vi "2.1 Interpret NMEA Sentence.vi"(11 "NMEA Sentence":string) -> ()   [LabVIEW 2011]
doc: "Interprets the NMEA 0813 sentences that we are using from our Airmar PB200 WeatherStation sensor.\nBy Jaime McCandless\nTODO: finish implementing NMEA sentences"
uses:
  <vilib>/regexp/Match Regular Expression.xnode
panel:
  out "Tab Control":enum32{"GPRMC", "GPGGA", "GPGLL"}(tab)
  out "UTC Time":timestamp
  out "Local Time":timestamp
  out "Lattitude (ddmm.mmmm)":dbl format="%_8g"
  out "Lattitude North/South":string
  out "Longitude (ddmm.mmmm)":dbl format="%_8g"
  out "Longitude East/West":string
  out "Speed over ground (knots)":dbl format="%_3g"
  out "Course over ground (degrees)":dbl format="%_4g"
  out "Magnetic Variation (degrees)":dbl format="%_4g"
  out "Variation East/West":string
  out "GPS (RMC) Data":T1 {"Course over ground (degrees)" format="%#.6g"; "Speed over ground (knots)" format="%#.6g"; "Magnetic Variation (degrees)" format="%#.6g"; "Longitude (ddmm.mmmm)" format="%#.6g"; "Lattitude (ddmm.mmmm)" format="%#.6g"}
  in  "UTC Time Zone":i32=-5
  out "GPS Data Valid?":bool
  out "UTC Time":timestamp
  out "Local Time":timestamp
  out "Lattitude (ddmm.mmmm)":dbl format="%_8g"
  out "Longitude (ddmm.mmmm)":dbl format="%_8g"
  out "Latitude North/South":string
  out "Longitude East/West":string
  in  "UTC Time Zone":i32=-5
  out "GPS Quality":T2(ring)
  out "GPS (GGA) Data":T3
  out "UTC Time":timestamp
  out "Local Time":timestamp
  out "Lattitude (ddmm.mmmm)":dbl format="%_8g"
  out "Lattitude North/South":string
  out "Longitude (ddmm.mmmm)":dbl format="%_8g"
  out "Longitude East/West":string
  in  "UTC Time Zone":i32=-5
  out "GPS Mode":string
  out "GPS Data Valid?":bool
  out "GPS (GLL) Data":T4
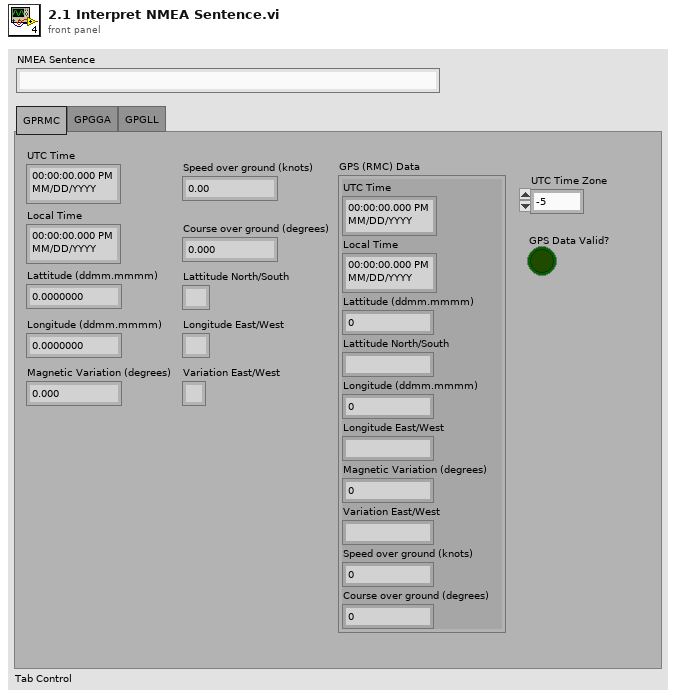
[diagram p1: front panel]
types:
  T1 = cluster{"UTC Time":timestamp, "Local Time":timestamp, "Lattitude (ddmm.mmmm)":dbl, "Lattitude North/South":string, "Longitude (ddmm.mmmm)":dbl, "Longitude East/West":string, "Magnetic Variation (degrees)":dbl, "Variation East/West":string, "Speed over ground (knots)":dbl, "Course over ground (degrees)":dbl}
  T2 = enum16{"Fix not available or invalid", "GPS SPS Mode, fix valid", "Differential GPS, SPS Mode, fix valid", "GPS PPS Mode, fix valid", "Real Time Kinematic (RTK)", "Float RTK", "Estimated (dead reckoning) Mode", "Manual Input Mode", "Simulator Mode"}
  T3 = cluster{"UTC Time":timestamp, "Local Time":timestamp, "Lattitude (ddmm.mmmm)":dbl, "Lattitude North/South":string, "Longitude (ddmm.mmmm)":dbl, "Longitude East/West":string, "GPS Quality":enum16{"Fix not available or invalid", "GPS SPS Mode, fix valid", "Differential GPS, SPS Mode, fix valid", "GPS PPS Mode, fix valid", "Real Time Kinematic (RTK)", "Float RTK", "Estimated (dead reckoning) Mode", "Manual Input Mode", "Simulator Mode"}}
  T4 = cluster{"UTC Time":timestamp, "Local Time":timestamp, "Lattitude (ddmm.mmmm)":dbl, "Lattitude North/South":string, "Longitude (ddmm.mmmm)":dbl, "Longitude East/West":string, "GPS Mode":string, "GPS Data Valid?":bool}
  T5 = cluster{"second":i32, "minute":i32, "hour":i32, "day of month":i32, "month":i32, "year":i32, "day of week":i32, "day of year":i32, "is DST":i32}
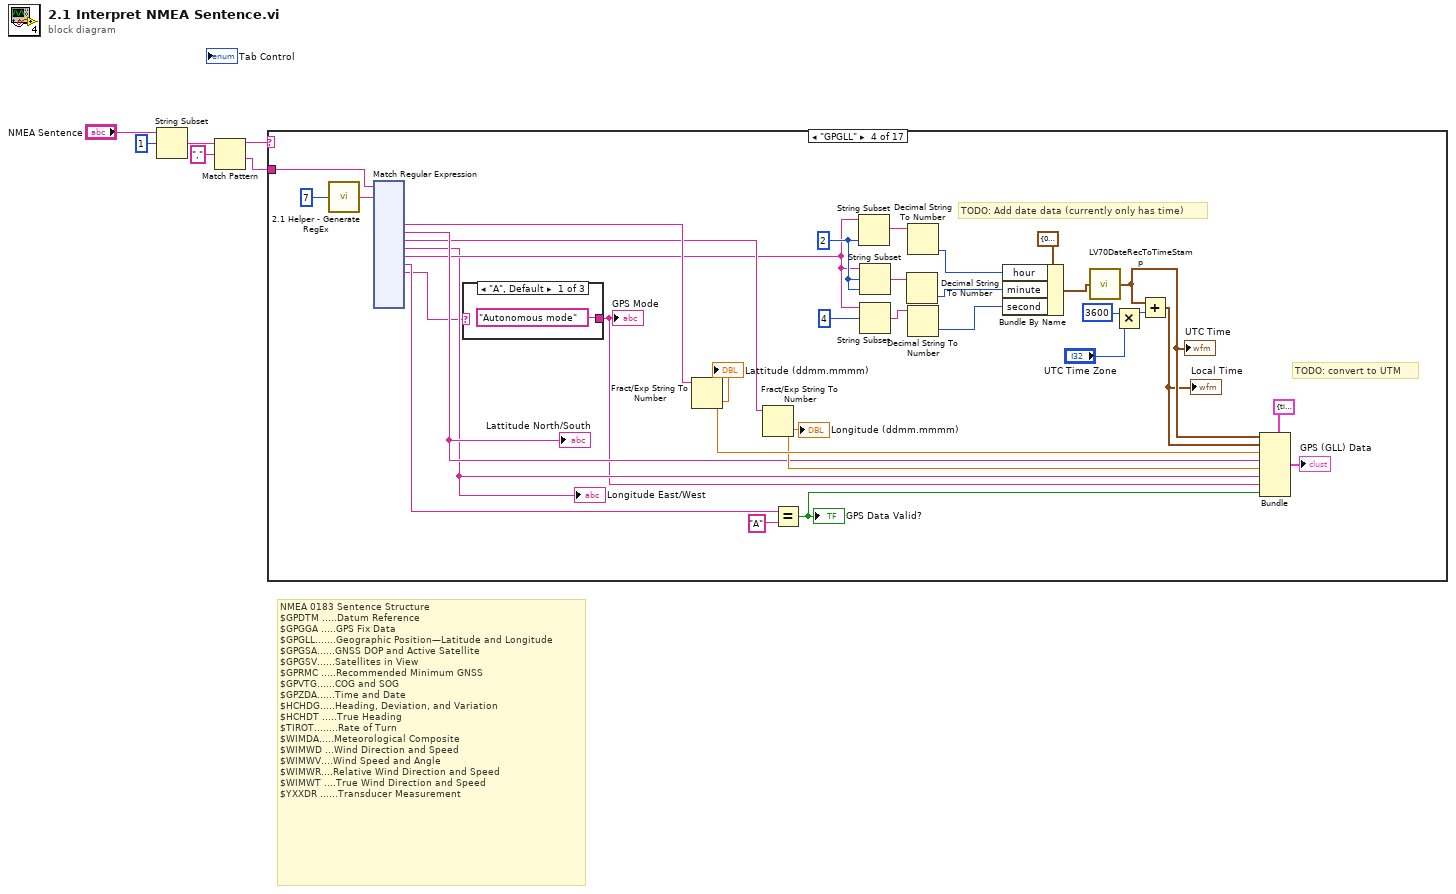
[diagram p0: block diagram]
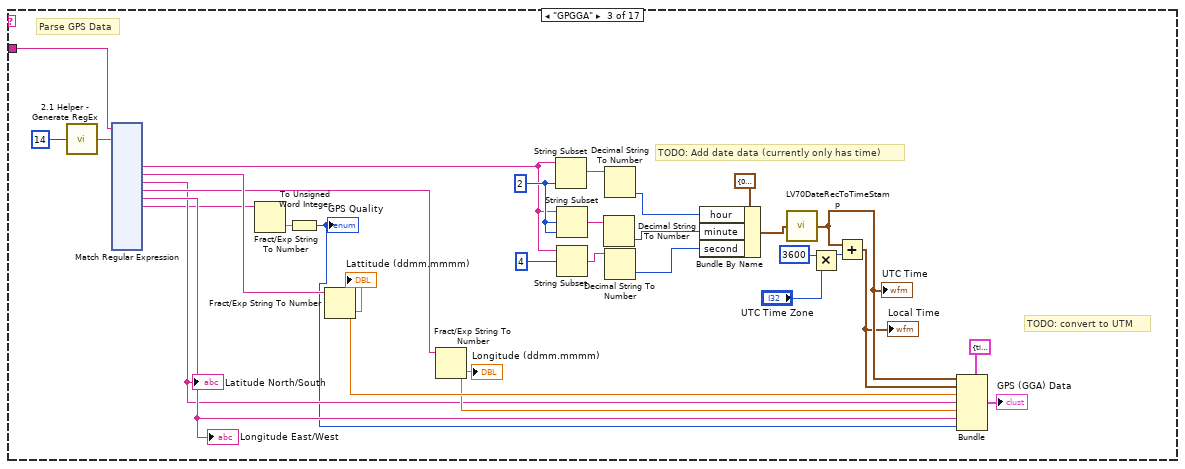
[diagram p4: hidden frame]
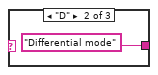
[diagram p5: hidden frame]
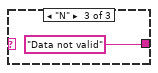
[diagram p6: hidden frame]
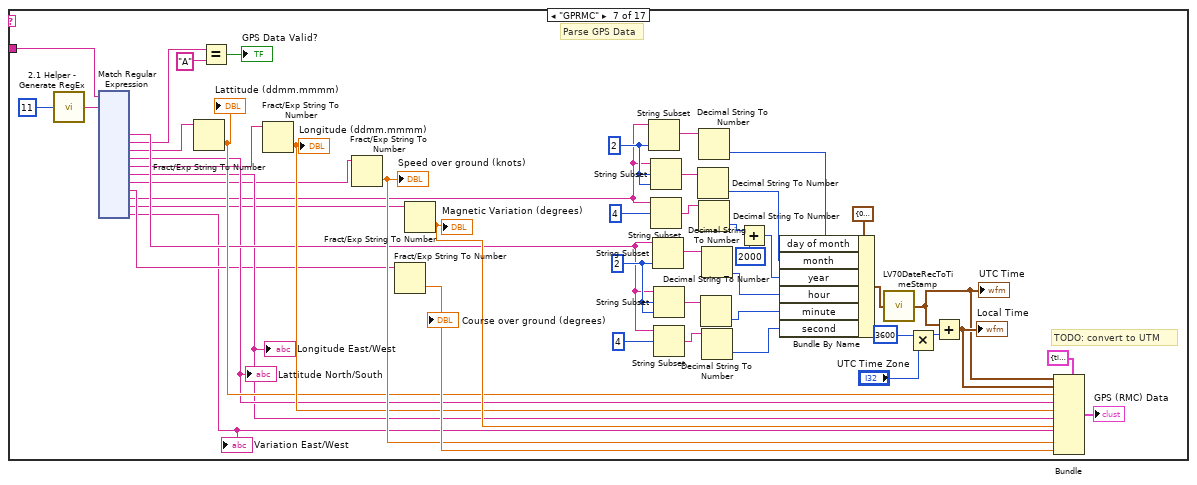
[diagram p9: hidden frame]
diagram:
  # "NMEA 0183 Sentence Structure\n$GPDTM .....Datum Reference\n$GPGGA .....GPS Fix Data\n$GPGLL.......Geographic Position—Latitude and Longitude\n$GPGSA......GNSS DOP and Active Satellite\n$GPGSV......Satellites in View\n$GPRMC .....Recommended Minimum GNSS\n$GPVTG......COG and SOG\n$GPZDA......Time and Date\n$HCHDG.....Heading, Deviation, and Variation\n$HCHDT .....True Heading\n$TIROT........Rate of Turn\n$WIMDA.....Meteorological Composite\n$WIMWD ...Wind Direction and Speed\n$WIMWV....Wind Speed and Angle\n$WIMWR....Relative Wind Direction and Speed\n$WIMWT ....True Wind Direction and Speed\n$YXXDR ......Transducer Measurement"
  n1 = String Subset(string="NMEA Sentence", offset (0)=1) -> (substring=w3:string)  [unwired: 1 in]
  n2 = Match Pattern(string=w3, regular expression=",") -> (before substring=w4:string, after substring=w5:string)  [unwired: 1 in, 2 out]
  n3 = case shown="\"GPGLL\"" w4 {
    tunnel: w5 -> [_ _ w34 w160 _ _ w330 _ _ _ _ _ _ _ _ _ _]
    frame "", Default {
    }
    frame "GPDTM" {
    }
    frame "GPGGA" {
      w29 = 2 ("length (rest)")
      # "TODO: convert to UTM"
      # "TODO: Add date data (currently only has time)"
      # "Parse GPS Data"
      n4 = call "2.1 Helper - Generate RegEx.vi"("# Datums"=14) -> ("RegEx"=w35:string)
      n5 = xnode "Match Regular Expression"("input string"=w34, "regular expression"=w35) -> ("submatch 1"=w9:string, "submatch 2"=w15:string, "submatch 3"=w12:string, "submatch 4"=w14:string, "submatch 5"=w13:string, "submatch 6"=w11:string)  [unwired: 4 in, 10 out]
      "Latitude North/South" <- w12
      "Longitude East/West" <- w13
      n6 = Fract/Exp String To Number(string=w11) -> (number=w10:dbl)  [unwired: 3 in, 1 out]
      n7 = To Unsigned Word Integer(number=w10) -> (unsigned 16bit integer=w8:u16)
      "GPS Quality" <- w8
      n8 = Fract/Exp String To Number(string=w15) -> (number=w18:dbl)  [unwired: 3 in, 1 out]
      "Lattitude (ddmm.mmmm)" <- w18
      n9 = Fract/Exp String To Number(string=w14) -> (number=w17:dbl)  [unwired: 3 in, 1 out]
      "Longitude (ddmm.mmmm)" <- w17
      n10 = String Subset(string=w9, length (rest)=w29) -> (substring=w33:string)  [unwired: 1 in]
      n11 = String Subset(string=w9, offset (0)=w29, length (rest)=w29) -> (substring=w27:string)
      n12 = String Subset(string=w9, offset (0)=4) -> (substring=w25:string)  [unwired: 1 in]
      n13 = Decimal String To Number(string=w27) -> (number=w28:i32)  [unwired: 2 in, 1 out]
      n14 = Decimal String To Number(string=w33) -> (number=w30:i32)  [unwired: 2 in, 1 out]
      n15 = Decimal String To Number(string=w25) -> (number=w24:i32)  [unwired: 2 in, 1 out]
      n16 = Bundle By Name(cluster=T5 {"second"=0, "minute"=0, "hour"=0, "day of month"=0, "month"=0, "year"=0, "day of week"=0, "day of year"=0, "is DST"=0} ("date time rec 2"), "hour"=w30, "minute"=w28, "second"=w24) -> (w32:T5)
      n17 = call <vilib>:"LV70DateRecToTimeStamp.vi"("date time rec"=w32) -> ("Time Stamp"=w20:timestamp)
      "UTC Time" <- w20
      n18 = Multiply(x=3600 ("number"), y="UTC Time Zone") -> (x*y=w21:i32)
      n19 = Add(x=w20, y=w21) -> (x+y=w19:timestamp)
      "Local Time" <- w19
      n20 = Bundle(cluster=T3 {"UTC Time"=timestamp(0 s since 1904-01-01), "Local Time"=timestamp(0 s since 1904-01-01), "Lattitude (ddmm.mmmm)"=0.0, "Lattitude North/South"="", "Longitude (ddmm.mmmm)"=0.0, "Longitude East/West"="", "GPS Quality"=enum."GPS SPS Mode, fix valid"} ("Cluster"), "UTC Time"=w20, "Local Time"=w19, "Lattitude (ddmm.mmmm)"=w18, "Lattitude North/South"=w12, "Longitude (ddmm.mmmm)"=w17, "Longitude East/West"=w13, "GPS Quality"=w8) -> (→"GPS (GGA) Data":T3)
    }
    frame "GPGLL" {
      w185 = 2 ("length (rest)")
      # "TODO: convert to UTM"
      # "TODO: Add date data (currently only has time)"
      n21 = call "2.1 Helper - Generate RegEx.vi"("# Datums"=7) -> ("RegEx"=w190:string)
      n22 = xnode "Match Regular Expression"("input string"=w160, "regular expression"=w190) -> ("submatch 1"=w171:string, "submatch 2"=w170:string, "submatch 3"=w169:string, "submatch 4"=w165:string, "submatch 5"=w168:string, "submatch 6"=w166:string, "submatch 7"=w164:string)  [unwired: 4 in, 9 out]
      "Lattitude North/South" <- w170
      "Longitude East/West" <- w165
      n23 = case shown="\"A\", Default" w164 {
        tunnel: ["Autonomous mode" "Differential mode" "Data not valid"] -> w161
        frame "A", Default {
        }
        frame "D" {
        }
        frame "N" {
        }
      }
      "GPS Mode" <- w161
      n24 = Fract/Exp String To Number(string=w171) -> (number=w174:dbl)  [unwired: 3 in, 1 out]
      "Lattitude (ddmm.mmmm)" <- w174
      n25 = Fract/Exp String To Number(string=w169) -> (number=w173:dbl)  [unwired: 3 in, 1 out]
      "Longitude (ddmm.mmmm)" <- w173
      n26 = Equal?(x=w166, y="A") -> (x = y?=w162:bool)
      "GPS Data Valid?" <- w162
      n27 = String Subset(string=w168, length (rest)=w185) -> (substring=w189:string)  [unwired: 1 in]
      n28 = String Subset(string=w168, offset (0)=w185, length (rest)=w185) -> (substring=w183:string)
      n29 = String Subset(string=w168, offset (0)=4) -> (substring=w181:string)  [unwired: 1 in]
      n30 = Decimal String To Number(string=w183) -> (number=w184:i32)  [unwired: 2 in, 1 out]
      n31 = Decimal String To Number(string=w189) -> (number=w186:i32)  [unwired: 2 in, 1 out]
      n32 = Decimal String To Number(string=w181) -> (number=w180:i32)  [unwired: 2 in, 1 out]
      n33 = Bundle By Name(cluster=T5 {"second"=0, "minute"=0, "hour"=0, "day of month"=0, "month"=0, "year"=0, "day of week"=0, "day of year"=0, "is DST"=0} ("date time rec 2"), "hour"=w186, "minute"=w184, "second"=w180) -> (w188:T5)
      n34 = call <vilib>:"LV70DateRecToTimeStamp.vi"("date time rec"=w188) -> ("Time Stamp"=w176:timestamp)
      "UTC Time" <- w176
      n35 = Multiply(x=3600 ("number"), y="UTC Time Zone") -> (x*y=w177:i32)
      n36 = Add(x=w176, y=w177) -> (x+y=w175:timestamp)
      "Local Time" <- w175
      n37 = Bundle(cluster=T4 {"UTC Time"=timestamp(0 s since 1904-01-01), "Local Time"=timestamp(0 s since 1904-01-01), "Lattitude (ddmm.mmmm)"=0.0, "Lattitude North/South"="", "Longitude (ddmm.mmmm)"=0.0, "Longitude East/West"="", "GPS Mode"="", "GPS Data Valid?"=FALSE} ("Cluster"), "UTC Time"=w176, "Local Time"=w175, "Lattitude (ddmm.mmmm)"=w174, "Lattitude North/South"=w170, "Longitude (ddmm.mmmm)"=w173, "Longitude East/West"=w165, "GPS Mode"=w161, "GPS Data Valid?"=w162) -> (→"GPS (GLL) Data":T4)
    }
    frame "GPGSA" {
    }
    frame "GPGSV" {
    }
    frame "GPRMC" {
      w350 = 2 ("length (rest)")
      w338 = 2 ("length (rest)")
      # "TODO: convert to UTM"
      # "Parse GPS Data"
      n38 = call "2.1 Helper - Generate RegEx.vi"("# Datums"=11) -> ("RegEx"=w318:string)
      n39 = xnode "Match Regular Expression"("input string"=w330, "regular expression"=w318) -> ("submatch 1"=w329:string, "submatch 2"=w328:string, "submatch 3"=w327:string, "submatch 4"=w326:string, "submatch 5"=w325:string, "submatch 6"=w324:string, "submatch 7"=w323:string, "submatch 8"=w322:string, "submatch 9"=w321:string, "submatch 10"=w320:string, "submatch 11"=w319:string)  [unwired: 4 in, 5 out]
      "Lattitude North/South" <- w326
      "Longitude East/West" <- w324
      "Variation East/West" <- w319
      n40 = Fract/Exp String To Number(string=w327) -> (number=w359:dbl)  [unwired: 3 in, 1 out]
      "Lattitude (ddmm.mmmm)" <- w359
      n41 = Equal?(x=w328, y="A") -> (x = y?=→"GPS Data Valid?":bool)
      n42 = Fract/Exp String To Number(string=w325) -> (number=w360:dbl)  [unwired: 3 in, 1 out]
      "Longitude (ddmm.mmmm)" <- w360
      n43 = Fract/Exp String To Number(string=w323) -> (number=w362:dbl)  [unwired: 3 in, 1 out]
      "Speed over ground (knots)" <- w362
      n44 = Fract/Exp String To Number(string=w322) -> (number=w363:dbl)  [unwired: 3 in, 1 out]
      "Course over ground (degrees)" <- w363
      n45 = Fract/Exp String To Number(string=w320) -> (number=w361:dbl)  [unwired: 3 in, 1 out]
      "Magnetic Variation (degrees)" <- w361
      n46 = String Subset(string=w321, length (rest)=w350) -> (substring=w351:string)  [unwired: 1 in]
      n47 = String Subset(string=w321, offset (0)=w350, length (rest)=w350) -> (substring=w349:string)
      n48 = String Subset(string=w321, offset (0)=4) -> (substring=w347:string)  [unwired: 1 in]
      n49 = String Subset(string=w329, length (rest)=w338) -> (substring=w334:string)  [unwired: 1 in]
      n50 = String Subset(string=w329, offset (0)=w338, length (rest)=w338) -> (substring=w340:string)
      n51 = String Subset(string=w329, offset (0)=4) -> (substring=w342:string)  [unwired: 1 in]
      n52 = Decimal String To Number(string=w349) -> (number=w353:i32)  [unwired: 2 in, 1 out]
      n53 = Decimal String To Number(string=w351) -> (number=w352:i32)  [unwired: 2 in, 1 out]
      n54 = Decimal String To Number(string=w347) -> (number=w354:i32)  [unwired: 2 in, 1 out]
      n55 = Decimal String To Number(string=w340) -> (number=w339:i32)  [unwired: 2 in, 1 out]
      n56 = Decimal String To Number(string=w334) -> (number=w337:i32)  [unwired: 2 in, 1 out]
      n57 = Decimal String To Number(string=w342) -> (number=w343:i32)  [unwired: 2 in, 1 out]
      n58 = Add(x=w354, y=2000) -> (x+y=w356:i32)
      n59 = Bundle By Name(cluster=T5 {"second"=0, "minute"=0, "hour"=0, "day of month"=0, "month"=0, "year"=0, "day of week"=0, "day of year"=0, "is DST"=0} ("date time rec"), "day of month"=w352, "month"=w353, "year"=w356, "hour"=w337, "minute"=w339, "second"=w343) -> (w335:T5)
      n60 = call <vilib>:"LV70DateRecToTimeStamp.vi"("date time rec"=w335) -> ("Time Stamp"=w357:timestamp)
      "UTC Time" <- w357
      n61 = Multiply(x=3600 ("number"), y="UTC Time Zone") -> (x*y=w346:i32)
      n62 = Add(x=w357, y=w346) -> (x+y=w358:timestamp)
      "Local Time" <- w358
      n63 = Bundle(cluster=T1 {"UTC Time"=timestamp(0 s since 1904-01-01), "Local Time"=timestamp(0 s since 1904-01-01), "Lattitude (ddmm.mmmm)"=0.0, "Lattitude North/South"="", "Longitude (ddmm.mmmm)"=0.0, "Longitude East/West"="", "Magnetic Variation (degrees)"=0.0, "Variation East/West"="", "Speed over ground (knots)"=0.0, "Course over ground (degrees)"=0.0} ("Cluster"), "UTC Time"=w357, "Local Time"=w358, "Lattitude (ddmm.mmmm)"=w359, "Lattitude North/South"=w326, "Longitude (ddmm.mmmm)"=w360, "Longitude East/West"=w324, "Magnetic Variation (degrees)"=w361, "Variation East/West"=w319, "Speed over ground (knots)"=w362, "Course over ground (degrees)"=w363) -> (→"GPS (RMC) Data":T1)
    }
    frame "GPVTG" {
    }
    frame "GPZDA" {
    }
    frame "HCHDG " {
    }
    frame "HCHDT" {
    }
    frame "TIROT" {
    }
    frame "WIMDA" {
    }
    frame "WIMWV" {
    }
    frame "WIMWR" {
    }
    frame "WIMWT" {
    }
    frame "YXXDR" {
    }
  }
